vi "VISA.Get Available Device Info.vi"(7 "Sort (F = Low to High)":bool caption="Auto", 8 "error in":errorcluster, 10 "Description Contains":string, 11 "Alias Contains":string) -> (0 "error out":errorcluster, 3 "Device Info":T1[](array[typedef]))   [LabVIEW 2018]
uses:
  <vilib>/Instr/_visa.llb/VISA Find Search Mode.ctl
  VISA.Device Info.ctl
panel:
  in  "VISA resource name":refnum<visa-resource-name>
  in  "PID":string="USB Serial Device"
  in  "VID":string="USB Serial Device"
  # "Get VISA Device Info"
  # "COM"
  # "USB Serial Device"
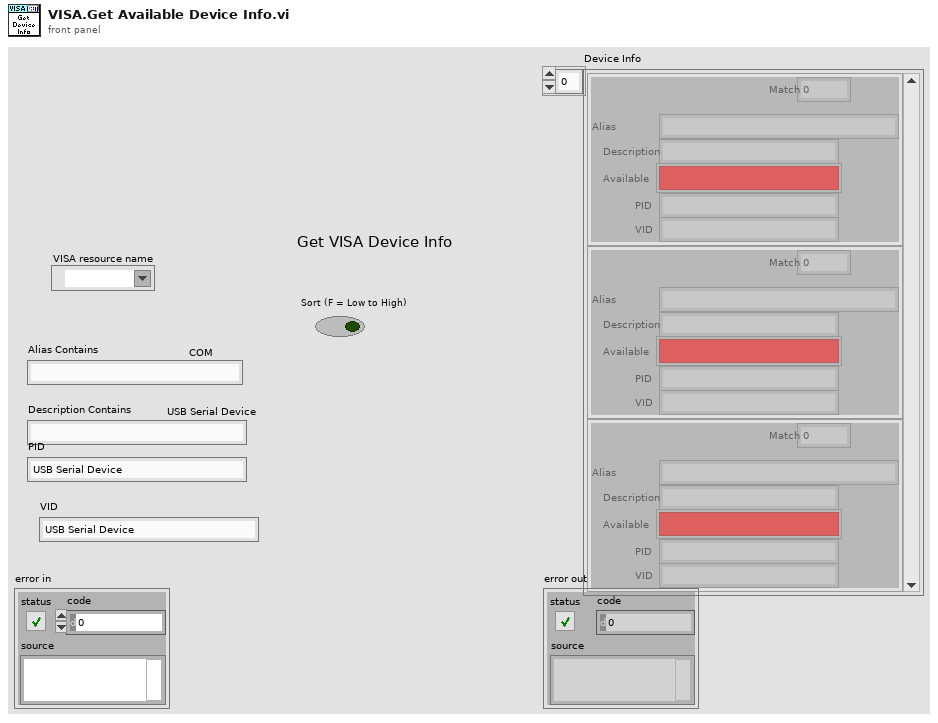
[diagram p1: front panel]
types:
  T1 = typedef "VISA.Device Info.ctl" = cluster{"Match":i32, "Alias":string, "Description":string, "Available":bool, "PID":string, "VID":string}
  T2 = typedef "VISA Find Search Mode.ctl" = u32
  T3 = cluster{"ID":string, "Type":string, "VID":string, "PID":string}[]
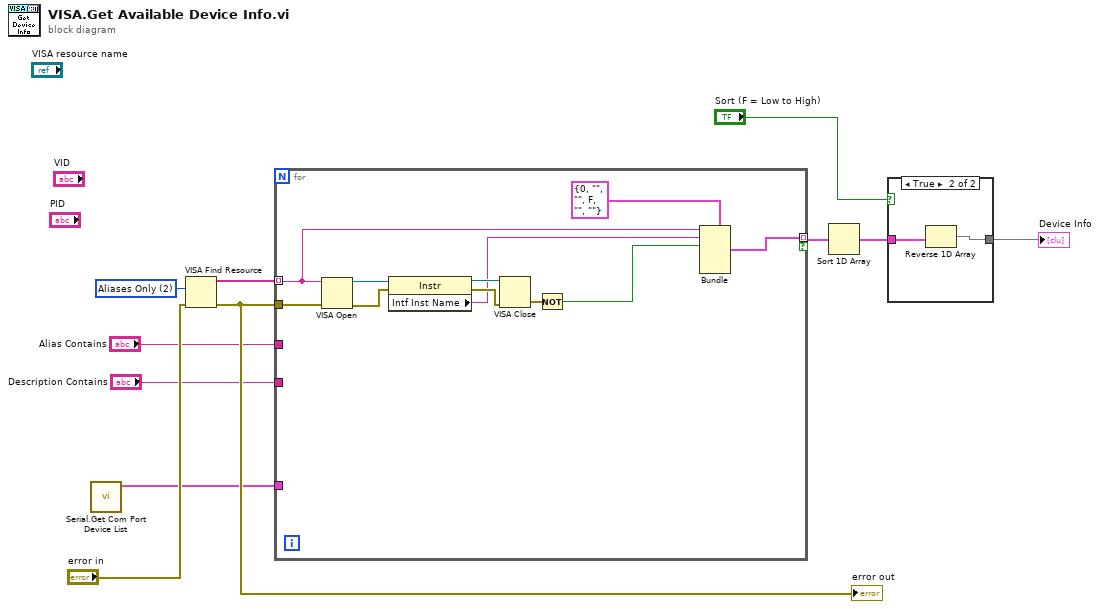
[diagram p0: block diagram]
diagram:
  w11 = T2 2 items=["Canonical Names Only"=0, "Aliases Only"=2, "Include Matching Aliases"=3, "Include All Aliases"=4] ("Search Mode")
  n1 = call "Serial.Get Com Port Device List.vi"() -> ("Ports"=w1:T3)  [unwired: 10 in, 1 out]
  n2 = VISA Find Resource(8:"error in", 10:w11) -> (0:w8:errorcluster, 3:w10:string[])  [unwired: 1 in, 1 out]
  "error out" <- w8
  n3 = for {
    tunnel: w10 -> [w13] mode=indexing
    tunnel: w8 -> [w22]
    tunnel: [w15] -> w5 mode=indexing if=_
    tunnel: "Alias Contains" -> [_]
    tunnel: "Description Contains" -> [_]
    tunnel: w1 -> [_]
    n4 = VISA Open(error in (no error)=w22, VISA resource name=w13) -> (VISA resource name=w21:refnum<visa-resource-name>, error out=w18:errorcluster)  [unwired: 3 in]
    n5 = property class="Instr"(reference=w21, error in=w18) -> (reference out=w20:refnum<visa-resource-name>, error out=w19:errorcluster, "Intf Inst Name"=w12:string)
    n6 = VISA Close(VISA resource name=w20, error in (no error)=w19) -> (error out=w17:errorcluster)
    n7 = Not(x=w17) -> (.not. x?=w16:bool)
    n8 = Bundle(cluster=T1 {"Match"=0, "Alias"="", "Description"="", "Available"=FALSE, "PID"="", "VID"=""} ("Device Info"), "Match"=w13, "Alias"=w12, "Description"=w16) -> (w15:T1)  [unwired: 3 in]
  }
  n9 = Sort 1D Array(array=w5) -> (sorted array=w3:T1[])
  n10 = case shown="True" "Sort (F = Low to High)" {
    tunnel: w3 -> [w23 w25]
    tunnel: [w23 w24] -> w2
    frame False {
    }
    frame True {
      n11 = Reverse 1D Array(array=w25) -> (reversed array=w24:T1[])
    }
  }
  "Device Info" <- w2
